vi "Autonomous Independent.vi"() -> ()   [LabVIEW 2012]
doc: "This VI is called when autonomous begins, and will automatically be terminated when autonomous ends. You can carry out timed or sensor driven robot movement independently without needing to return to the caller."
uses:
  Robot Global Data.vi
  <vilib>/Rock Robotics/WPI/RobotDrive/WPI_RobotDriveGetSetRefNum.vi
  <vilib>/Rock Robotics/WPI/Joystick/WPI_JoystickGetSetRefNum.vi
  Documents/LabVIEW Data/No Wayne Drive/wayne drive.vi
panel:
  in  "Distance 3":dbl=200.0
  in  "Distance 2":dbl=200.0
  in  "Distance":dbl=200.0
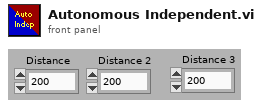
[diagram p1: front panel]
types:
  T1 = typedef "WPI_RobotDriveDevRef.ctl" = cluster{"DevStatus":errorcluster, "Motors[]":T2[], "Square Inputs":bool, "Max Output":dbl, "Isochronous":bool}
  T2 = typedef "WPI_MotorControlDeviceRef.ctl" = cluster{"DeviceStatus":errorcluster, "Type":enum16{"PWM", "CAN"}, "PWM":cluster{"Digital Module":T3, "PWM Channel":T4, "DeadBand":T5}, "CAN":cluster{"Device Number":u8, "Control Mode":T6, "Semaphore":T7, "Max Vout":dbl}, "Invert":bool, "TransformRef":T8, "InvTransformRef":T8}
  T3 = typedef "FPGA_TypedefDigitalModule.ctl" = enum16{"Digital Module 1", "Digital Module 2"}
  T4 = typedef "FPGA_DIOPWMChannel.ctl" = enum8{"PWM 1", "PWM 2", "PWM 3", "PWM 4", "PWM 5", "PWM 6", "PWM 7", "PWM 8", "PWM 9", "PWM 10", "Invalid"}
  T5 = typedef "WPI_PWMDeadband.ctl" = cluster{"Name":string, "maxPositivePwm":i32, "minPositivePwm":i32, "centerPwm":i32, "maxNegativePwm":i32, "minNegativePwm":i32, "angularRange":u16}
  T6 = typedef "WPI_CANJaguar_ControlMode.ctl" = enum8{"Percent VBus", "Current", "Speed", "Position", "Voltage"}
  T7 = typedef "Semaphore RefNum" = refnum<k1>
  T8 = typedef "WPI_PWMTransform_ConPane.ctl" = refnum<vi>
  T9 = typedef "WPI_JoystickDevRef.ctl" = cluster{"Device":T10}
  T10 = typedef "WPI_JoystickDeviceEnum.ctl" = enum16{"USB 1", "USB 2", "USB 3", "USB 4", "Kinect 1", "Kinect 2"}
  T11 = cluster{"axis 1 (x)":dbl, "axis 2 (y)":dbl, "axis 3 (throttle)":dbl, "axis 4":dbl, "axis 5":dbl, "axis 6":dbl}
  T12 = typedef "WPI_EncoderDevRef.ctl" = cluster{"DevStatus":errorcluster, "EncoderIndex":T13, "CounterIndex":T14, "DistancePerCount":dbl, "Decoding Type":T15}
  T13 = typedef "FPGA_EncoderIdx.ctl" = enum8{"Enc 0", "Enc 1", "Enc 2", "Enc 3", "Invalid"}
  T14 = typedef "FPGA_CounterCtrSystemIndex.ctl" = enum8{"Ctr 0", "Ctr 1", "Ctr 2", "Ctr 3", "Ctr 4", "Ctr 5", "Ctr 6", "Ctr 7", "Invalid"}
  T15 = typedef "WPI_EncoderType.ctl" = enum16{"1x", "2x", "4x"}
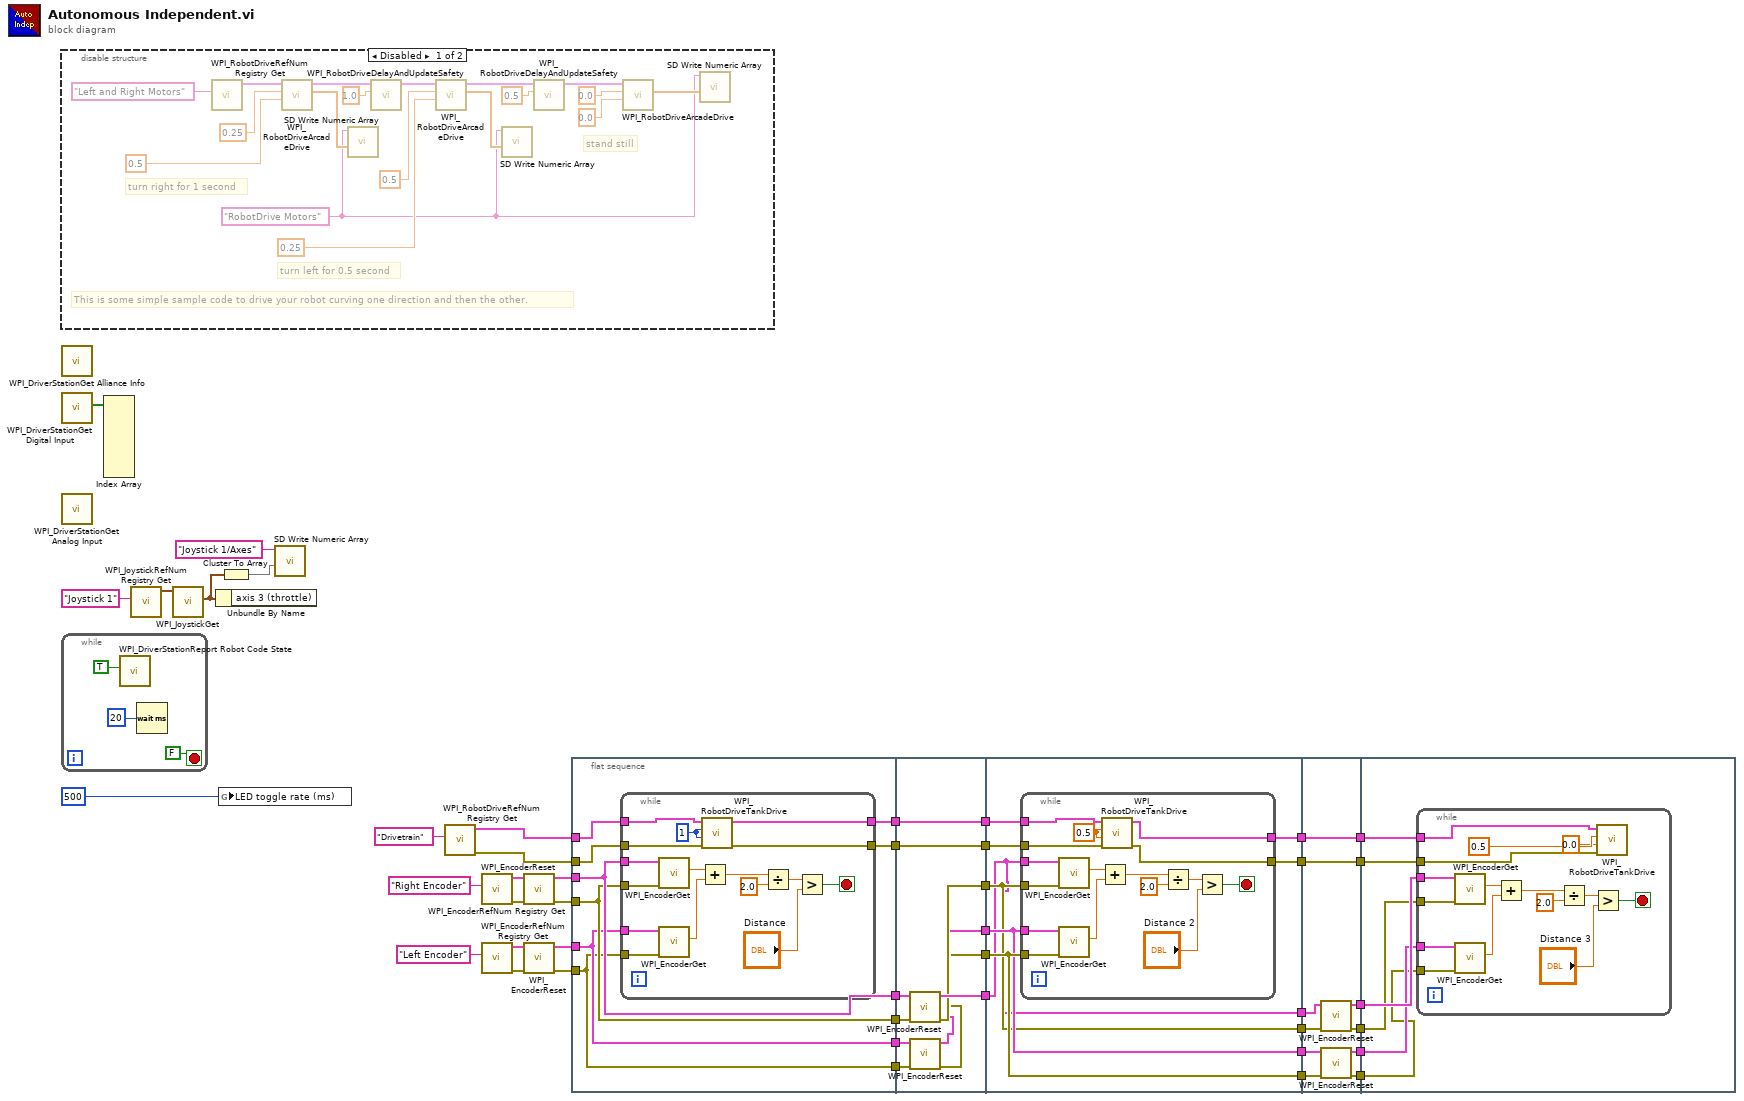
[diagram p0: block diagram]
diagram:
  n1 = disable-structure shown="Disabled" {
    frame Disabled {
      w45 = "RobotDrive Motors" ("Name")
      # "This is some simple sample code to drive your robot curving one direction and then the other."
      # "stand still"
      # "turn left for 0.5 second"
      # "turn right for 1 second"
      n2 = call <vilib>:"WPI_RobotDriveRefNum Registry Get.vi"("refnum name"="Left and Right Motors") -> ("RobotDriveDevRef"=w49:T1)  [unwired: 1 in, 9 out]
      n3 = call-poly <vilib>:"WPI_RobotDriveArcadeDrive.vi"("Y axis value"=0.5 ("X axis value"), "X axis value"=0.25, "RobotDriveDevRef"=w49) -> ("Motor Values"=w48:dbl[], "RobotDriveDevRef"=w56:T1)  [unwired: 1 in, 6 out]
      n4 = call <vilib>:"SD Write Numeric Array.vi"("Numeric Array"=w48, "Name"=w45) -> ()  [unwired: 8 in, 2 out]
      n5 = call <vilib>:"WPI_RobotDriveDelayAndUpdateSafety.vi"("Delay (s)"=1.0, "RobotDriveDevRef"=w56) -> ("RobotDriveDevRef 2"=w55:T1)  [unwired: 8 in, 1 out]
      n6 = call-poly <vilib>:"WPI_RobotDriveArcadeDrive.vi"("Y axis value"=0.25 ("X axis value"), "X axis value"=0.5, "RobotDriveDevRef"=w55) -> ("Motor Values"=w47:dbl[], "RobotDriveDevRef"=w54:T1)  [unwired: 1 in, 6 out]
      n7 = call <vilib>:"SD Write Numeric Array.vi"("Numeric Array"=w47, "Name"=w45) -> ()  [unwired: 8 in, 2 out]
      n8 = call <vilib>:"WPI_RobotDriveDelayAndUpdateSafety.vi"("Delay (s)"=0.5, "RobotDriveDevRef"=w54) -> ("RobotDriveDevRef 2"=w53:T1)  [unwired: 8 in, 1 out]
      n9 = call-poly <vilib>:"WPI_RobotDriveArcadeDrive.vi"("Y axis value"=0.0 ("X axis value"), "X axis value"=0.0, "RobotDriveDevRef"=w53) -> ("Motor Values"=w46:dbl[])  [unwired: 1 in, 7 out]
      n10 = call <vilib>:"SD Write Numeric Array.vi"("Numeric Array"=w46, "Name"=w45) -> ()  [unwired: 8 in, 2 out]
    }
    frame Enabled {
    }
  }
  n11 = call <vilib>:"WPI_DriverStationGet Alliance Info.vi"() -> ()  [unwired: 12 out]
  n12 = call <vilib>:"WPI_DriverStationGet Digital Input.vi"() -> ("Driver Station Digital Input (1-8)"=w44:bool[])  [unwired: 11 out]
  n13 = call <vilib>:"WPI_DriverStationGet Analog Input.vi"() -> ()  [unwired: 12 out]
  n14 = while {
    stop <- FALSE stop-if-true
    n15 = call <vilib>:"WPI_DriverStationReport Robot Code State.vi"("Autonomous"=TRUE) -> ()  [unwired: 10 in, 1 out]
    n16 = Wait (ms)(milliseconds to wait=u32 20) -> ()  [unwired: 1 out]
  }
  n17 = Index Array(array=w44) -> ()  [unwired: 8 in, 8 out]
  n18 = call <vilib>:"WPI_JoystickRefNum Registry Get.vi"("refnum name"="Joystick 1") -> ("JoystickDevRef"=w42:T9)  [unwired: 1 in, 9 out]
  n19 = call <vilib>:"WPI_JoystickGet.vi"("JoystickDevRef"=w42) -> ("Axes"=w39:T11)  [unwired: 1 in, 5 out]
  n20 = Unbundle By Name(w39) -> ()  [unwired: 1 out]
  n21 = global write "Robot Global Data.vi" "LED toggle rate (ms)"(u32 500 ("LED ms toggle rate")) -> ()
  n22 = Cluster To Array(cluster=w39) -> (array=w40:dbl[])
  n23 = call <vilib>:"SD Write Numeric Array.vi"("Numeric Array"=w40, "Name"="Joystick 1/Axes") -> ()  [unwired: 8 in, 2 out]
  n24 = call <vilib>:"WPI_RobotDriveRefNum Registry Get.vi"("refnum name"="Drivetrain") -> ("error out"=w24:errorcluster, "RobotDriveDevRef"=w25:T1)  [unwired: 9 in]
  n25 = call <vilib>:"WPI_EncoderRefNum Registry Get.vi"("refnum name"="Right Encoder") -> ("error out"=w33:errorcluster, "EncoderDevRef"=w32:T12)  [unwired: 9 in]
  n26 = call <vilib>:"WPI_EncoderRefNum Registry Get.vi"("refnum name"="Left Encoder") -> ("error out"=w31:errorcluster, "EncoderDevRef"=w30:T12)  [unwired: 9 in]
  n27 = call <vilib>:"WPI_EncoderReset.vi"("error in (no error)"=w33, "EncoderDevRef"=w32) -> ("error out"=w28:errorcluster, "EncoderDevRef"=w29:T12)  [unwired: 8 in]
  n28 = call <vilib>:"WPI_EncoderReset.vi"("error in (no error)"=w31, "EncoderDevRef"=w30) -> ("error out"=w26:errorcluster, "EncoderDevRef"=w27:T12)  [unwired: 8 in]
  n29 = flat-sequence {
    tunnel: w29 -> [w71]
    tunnel: w28 -> [w70]
    tunnel: w27 -> [w69]
    tunnel: w26 -> [w68]
    tunnel: w25 -> [w73]
    tunnel: w24 -> [w72]
    tunnel: [w71] -> w37
    tunnel: [w70] -> w36
    tunnel: [w69] -> w35
    tunnel: [w68] -> w34
    tunnel: [w67] -> w20
    tunnel: [w66] -> w17
    tunnel: w37 -> [w99]
    tunnel: w36 -> [w98]
    tunnel: w35 -> [w97]
    tunnel: w34 -> [w96]
    tunnel: w20 -> [w95]
    tunnel: [w95] -> w19
    tunnel: [w94] -> w18
    tunnel: w17 -> [w94]
    tunnel: [w93] -> w16
    tunnel: [w92] -> w15
    tunnel: [w91] -> w14
    tunnel: [w90] -> w13
    tunnel: w19 -> [w107]
    tunnel: w18 -> [w106]
    tunnel: w16 -> [w100]
    tunnel: w15 -> [w101]
    tunnel: w14 -> [w102]
    tunnel: w13 -> [w103]
    tunnel: [w105] -> w11
    tunnel: [w104] -> w9
    tunnel: [w103] -> w8
    tunnel: [w102] -> w7
    tunnel: [w101] -> w6
    tunnel: [w100] -> w5
    tunnel: [w133] -> w12
    tunnel: w11 -> [w133]
    tunnel: [w132] -> w10
    tunnel: w9 -> [w132]
    tunnel: w8 -> [w131]
    tunnel: w7 -> [w130]
    tunnel: w6 -> [w129]
    tunnel: w5 -> [w128]
    tunnel: [w127] -> w4
    tunnel: [w126] -> w3
    tunnel: [w125] -> w2
    tunnel: [w124] -> w1
    tunnel: w12 -> [w139]
    tunnel: w10 -> [w138]
    tunnel: w4 -> [w137]
    tunnel: w3 -> [w136]
    tunnel: w2 -> [w135]
    tunnel: w1 -> [w134]
    frame #0 {
      n30 = while {
        tunnel: w71 -> [w89]
        tunnel: w70 -> [w88]
        tunnel: w69 -> [w87]
        tunnel: w68 -> [w86]
        tunnel: w73 -> [w81]
        tunnel: w72 -> [w80]
        tunnel: [w75] -> w67
        tunnel: [w74] -> w66
        stop <- w79 stop-if-true
        w76 = 1
        n31 = call <vilib>:"WPI_EncoderGet.vi"("error in (no error)"=w88, "EncoderDevRef"=w89) -> ("Distance"=w78:dbl)  [unwired: 4 in, 5 out]
        n32 = call <vilib>:"WPI_EncoderGet.vi"("error in (no error)"=w86, "EncoderDevRef"=w87) -> ("Distance"=w77:dbl)  [unwired: 4 in, 5 out]
        n33 = Add(x=w78, y=w77) -> (x+y=w84:dbl)
        n34 = call <vilib>:"WPI_RobotDriveTankDrive.vi"("error in (no error)"=w80, "Right axis value"=w76, "Left axis value"=w76, "RobotDriveDevRef"=w81) -> ("error out"=w74:errorcluster, "RobotDriveDevRef"=w75:T1)  [unwired: 5 in, 1 out]
        n35 = Divide(x=w84, y=2.0) -> (x/y=w82:dbl)
        n36 = Greater?(x=w82, y="Distance") -> (0:w79:bool)
      }
    }
    frame #1 {
      n37 = call <vilib>:"WPI_EncoderReset.vi"("error in (no error)"=w98, "EncoderDevRef"=w99) -> ("error out"=w92:errorcluster, "EncoderDevRef"=w93:T12)  [unwired: 8 in]
      n38 = call <vilib>:"WPI_EncoderReset.vi"("error in (no error)"=w96, "EncoderDevRef"=w97) -> ("error out"=w90:errorcluster, "EncoderDevRef"=w91:T12)  [unwired: 8 in]
    }
    frame #2 {
      n39 = while {
        tunnel: w100 -> [w123]
        tunnel: w101 -> [w122]
        tunnel: w102 -> [w121]
        tunnel: w103 -> [w120]
        tunnel: w107 -> [w115]
        tunnel: w106 -> [w114]
        tunnel: [w109] -> w105
        tunnel: [w108] -> w104
        stop <- w113 stop-if-true
        w110 = 0.5
        n40 = call <vilib>:"WPI_EncoderGet.vi"("error in (no error)"=w122, "EncoderDevRef"=w123) -> ("Distance"=w112:dbl)  [unwired: 4 in, 5 out]
        n41 = call <vilib>:"WPI_EncoderGet.vi"("error in (no error)"=w120, "EncoderDevRef"=w121) -> ("Distance"=w111:dbl)  [unwired: 4 in, 5 out]
        n42 = Add(x=w112, y=w111) -> (x+y=w118:dbl)
        n43 = call <vilib>:"WPI_RobotDriveTankDrive.vi"("error in (no error)"=w114, "Right axis value"=w110, "Left axis value"=w110, "RobotDriveDevRef"=w115) -> ("error out"=w108:errorcluster, "RobotDriveDevRef"=w109:T1)  [unwired: 5 in, 1 out]
        n44 = Divide(x=w118, y=2.0) -> (x/y=w116:dbl)
        n45 = Greater?(x=w116, y="Distance 2") -> (0:w113:bool)
      }
    }
    frame #3 {
      n46 = call <vilib>:"WPI_EncoderReset.vi"("error in (no error)"=w129, "EncoderDevRef"=w128) -> ("error out"=w126:errorcluster, "EncoderDevRef"=w127:T12)  [unwired: 8 in]
      n47 = call <vilib>:"WPI_EncoderReset.vi"("error in (no error)"=w131, "EncoderDevRef"=w130) -> ("error out"=w124:errorcluster, "EncoderDevRef"=w125:T12)  [unwired: 8 in]
    }
    frame #4 {
      n48 = while {
        tunnel: w137 -> [w154]
        tunnel: w136 -> [w153]
        tunnel: w135 -> [w152]
        tunnel: w134 -> [w141]
        tunnel: w139 -> [w147]
        tunnel: w138 -> [w146]
        stop <- w145 stop-if-true
        n49 = call <vilib>:"WPI_EncoderGet.vi"("error in (no error)"=w153, "EncoderDevRef"=w154) -> ("Distance"=w144:dbl)  [unwired: 4 in, 5 out]
        n50 = call <vilib>:"WPI_EncoderGet.vi"("error in (no error)"=w141, "EncoderDevRef"=w152) -> ("Distance"=w143:dbl)  [unwired: 4 in, 5 out]
        n51 = Add(x=w144, y=w143) -> (x+y=w150:dbl)
        n52 = Divide(x=w150, y=2.0) -> (x/y=w148:dbl)
        n53 = Greater?(x=w148, y="Distance 3") -> (0:w145:bool)
        n54 = call <vilib>:"WPI_RobotDriveTankDrive.vi"("error in (no error)"=w146, "Right axis value"=0.0, "Left axis value"=0.5, "RobotDriveDevRef"=w147) -> ()  [unwired: 5 in, 3 out]
      }
    }
  }
